vi "Read Handler.vi"(8 "error in (no error)":errorcluster, 11 "Logger in":refnum<class "Logger.lvclass">) -> (0 "error out":errorcluster, 2 "Handler":refnum<class "Formatting Handler.lvclass">, 3 "Logger out":refnum<class "Logger.lvclass">)   [LabVIEW 2018, in "GLog.lvlib" / "Logger.lvclass"]
uses:
  <vilib>/NQE/GLog/src/api/logger_class/Logger.lvclass
  <vilib>/NQE/GLog/src/api/extension/formatting_handler_interface/Formatting Handler.lvclass
  <vilib>/NQE/GLog/src/api/logger_class/Logger.lvclass/Logger.ctl
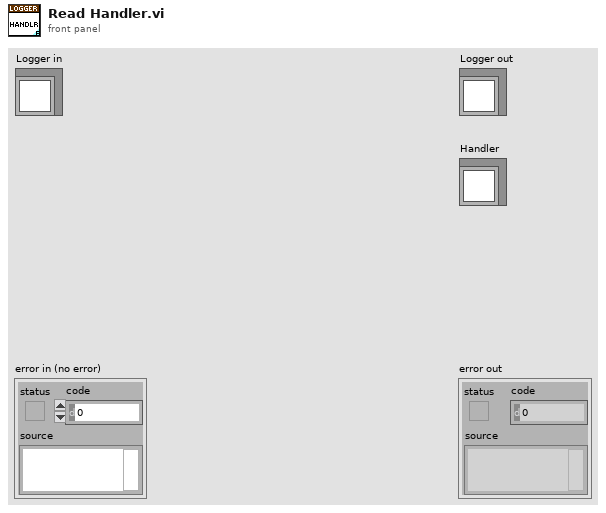
[diagram p1: front panel]
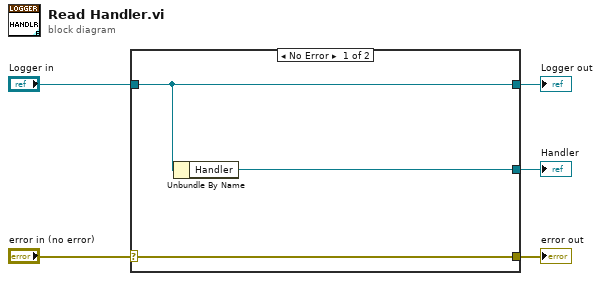
[diagram p0: block diagram]
diagram:
  n1 = case shown="No Error" "error in (no error)" {
    selector: "error in (no error)" -> [w8 w9]
    tunnel: [w8 w9] -> w4
    tunnel: [w7 w10] -> w2
    tunnel: "Logger in" -> [w7 w10]
    tunnel: [w6 _] -> w1
    frame No Error {
      n2 = Unbundle By Name(w7) -> ("Handler"=w6:refnum<class "Formatting Handler.lvclass">)
    }
    frame Error {
    }
  }
  "error out" <- w4
  "Logger out" <- w2
  "Handler" <- w1
